vi "Format Excluded Tests on Items.vi"(0 "excluded tests on items":T1(array[cluster])) -> (4 "formatted string":string)   [LabVIEW 2020]
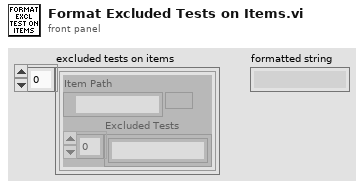
[diagram p1: front panel]
types:
  T1 = cluster{"Item Path":path, "Excluded Tests":string[]}[]
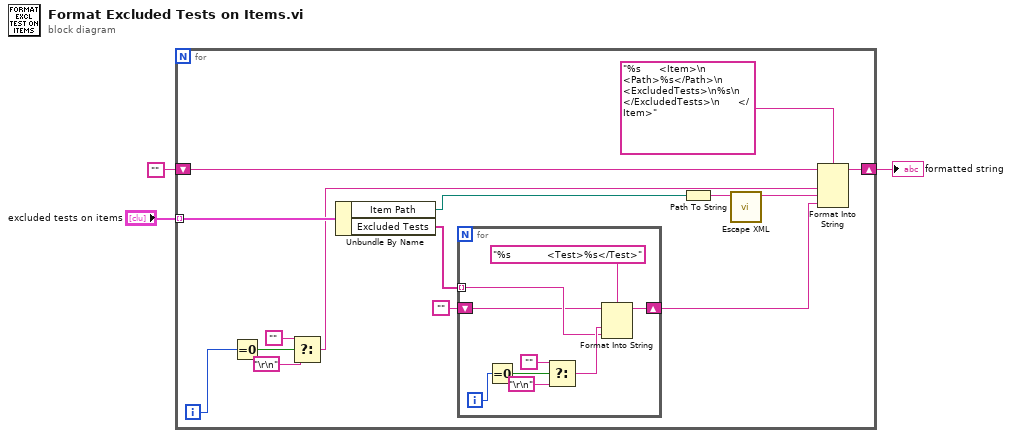
[diagram p0: block diagram]
diagram:
  n1 = for {
    tunnel: "excluded tests on items" -> [w18] mode=indexing
    shift-right: [w16] -> w3
    shift-left: "" -> [w17]
    i -> [w8]
    n2 = Equal To 0?(x=w8) -> (x = 0?=w9:bool)
    n3 = Select(t="", s=w9, f="\r\n") -> (s? t:f=w7:string)
    n4 = Unbundle By Name(w18) -> ("Item Path"=w5:path, "Excluded Tests"=w15:string[])
    n5 = for {
      tunnel: w15 -> [w20] mode=indexing
      shift-right: [w23] -> w12
      shift-left: "" -> [w19]
      i -> [w24]
      n6 = Equal To 0?(x=w24) -> (x = 0?=w27:bool)
      n7 = Select(t="", s=w27, f="\r\n") -> (s? t:f=w21:string)
      n8 = Format Into String(format string="%s            <Test>%s</Test>", initial string=w19, w21, w20) -> (resulting string=w23:string)  [unwired: 1 in, 1 out]
    }
    n9 = Path To String(path=w5) -> (string=w6:string)
    n10 = call <vilib>:"Escape XML.vi"("XML String In"=w6) -> ("XML String Out"=w4:string)  [unwired: 9 in, 1 out]
    n11 = Format Into String(format string="%s      <Item>\n         <Path>%s</Path>\n         <ExcludedTests>\n%s\n         </ExcludedTests>\n      </Item>", initial string=w17, w7, w4, w12) -> (resulting string=w16:string)  [unwired: 1 in, 1 out]
  }
  "formatted string" <- w3
